vi "LoadConfig.vi"(8 "error in (no error)":errorcluster, 9 "AC Config":T1={"Board 1 alias"="192.168.1.110", "Board 1 Enable"=FALSE, "Board 2 alias"="192.168.1.110", "Board 2 Enable"=FALSE}, 11 "ArrayController in":refnum<class "ArrayController.lvclass">) -> (0 "error out":errorcluster, 3 "ArrayController out":refnum<class "ArrayController.lvclass">)   [LabVIEW 2018, in "ArrayController.lvclass"]
doc: "Array Controller Com properties\nLocation of 64 Module setup files, one for horizontal polarization, one for vertical"
uses:
  ArrayController.lvclass
  ACConfig.ctl
  ArrayController.lvclass/ArrayController.ctl
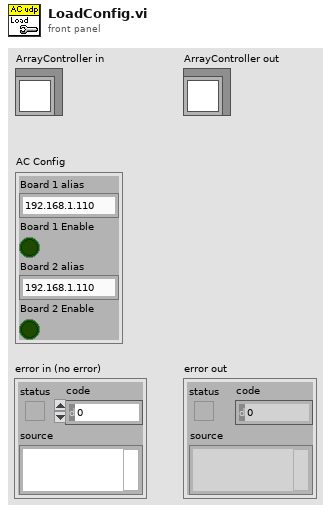
[diagram p1: front panel]
types:
  T1 = typedef "ACConfig.ctl" = cluster{"Board 1 alias":string, "Board 1 Enable":bool, "Board 2 alias":string, "Board 2 Enable":bool}
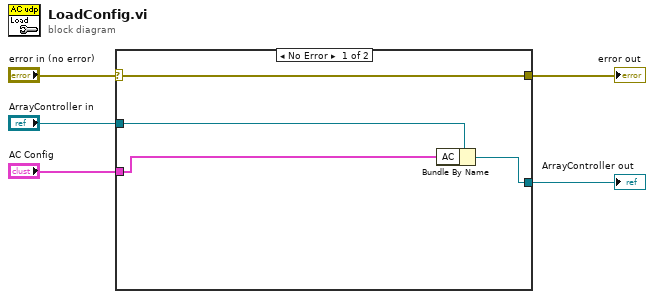
[diagram p0: block diagram]
diagram:
  n1 = case shown="No Error" "error in (no error)" {
    selector: "error in (no error)" -> [w9 w11]
    tunnel: [w9 w11] -> w4
    tunnel: [w6 w10] -> w2
    tunnel: "ArrayController in" -> [w7 w10]
    tunnel: "AC Config" -> [w8 _]
    frame No Error {
      n2 = Bundle By Name(cluster=w7, "AC"=w8) -> (w6:refnum<class "ArrayController.lvclass">)
    }
    frame Error {
    }
  }
  "error out" <- w4
  "ArrayController out" <- w2
